vi "Run Tests in Test Case.vi"(8 "error in (no error)":errorcluster, 10 "Test Case":refnum<class "LUnit Test Case.lvclass">, 11 "Slave Test Runner In":refnum<class "Slave Test Runner.lvclass">) -> (0 "error out":errorcluster, 2 "Test Case out":refnum<class "LUnit Test Case.lvclass">, 3 "Slave Test Runner Out":refnum<class "Slave Test Runner.lvclass">)   [LabVIEW 2020, in "Slave Test Runner.lvclass"]
doc: "Run Methods in Test Case."
uses:
  Slave Test Runner.lvclass
  Test Case/LUnit Test Case.lvclass
  Test Case/LUnit Test Case.lvclass/LUnit Test Case.ctl
  Result Classes/Method Result/Method Result.lvclass/Method Result.ctl
  Result Classes/Test Case Result/Test Case Result.lvclass/Test Case Result.ctl
  Slave Test Runner.lvclass/Slave Test Runner.ctl
  Result Collector/Result Collector.lvclass/Result Collector.ctl
  Test Case/Private/SubVIs/Pre Allocate Method Results.vi
  Test Case/Public/Accessors/Read Enabled Test Methods.vi
  Shuffle Test Methods.vi/2fc74b80-6deb-4f17-a78e-34401938511c.vi
  Result Classes/Test Case Result/Community/Handle Error.vi
  Result Classes/Test Case Result/Community/Set Method End Time.vi
  Result Classes/Test Case Result/Public/Accessors/Read Method Results.vi
  Result Collector/Public/API/Collect Method Results.vi
  Result Collector/Public/API/Collect Case Result.vi
  Test Case/Private/SubVIs/Read Test Case Name.vi
  Result Classes/Test Case Result/Community/Preallocate Method Results.vi
  Result Classes/Method Result/Public/Read Status.vi
  Result Classes/Method Result/Community/Accessors/Generate Error.vi
  Result Classes/Method Result/Community/Accessors/Write Execution time.vi
  Result Classes/Method Result/Community/Accessors/Write Test Method Name.vi
  Result Classes/Method Result/Community/Accessors/Write Test Case.vi
  <vilib>/Utility/LVClass/Get LV Class Name.vi
  <vilib>/Utility/semaphor.llb/Obtain Semaphore Reference.vi
  <vilib>/Utility/error.llb/Error Cluster From Error Code.vi
  <vilib>/Utility/semaphor.llb/Release Semaphore Reference.vi
  Result Classes/Test Case Result/Test Case Result.lvclass
  Result Classes/Method Result/Method Result.lvclass
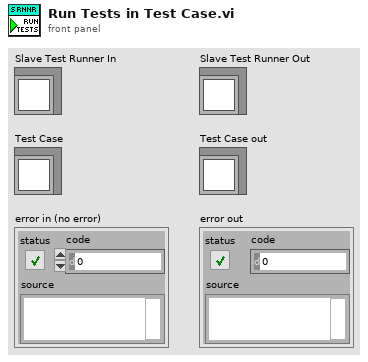
[diagram p1: front panel]
types:
  T1 = enum16{"Setup Error", "Teardown Error", "Broken", "Test Method Error"}
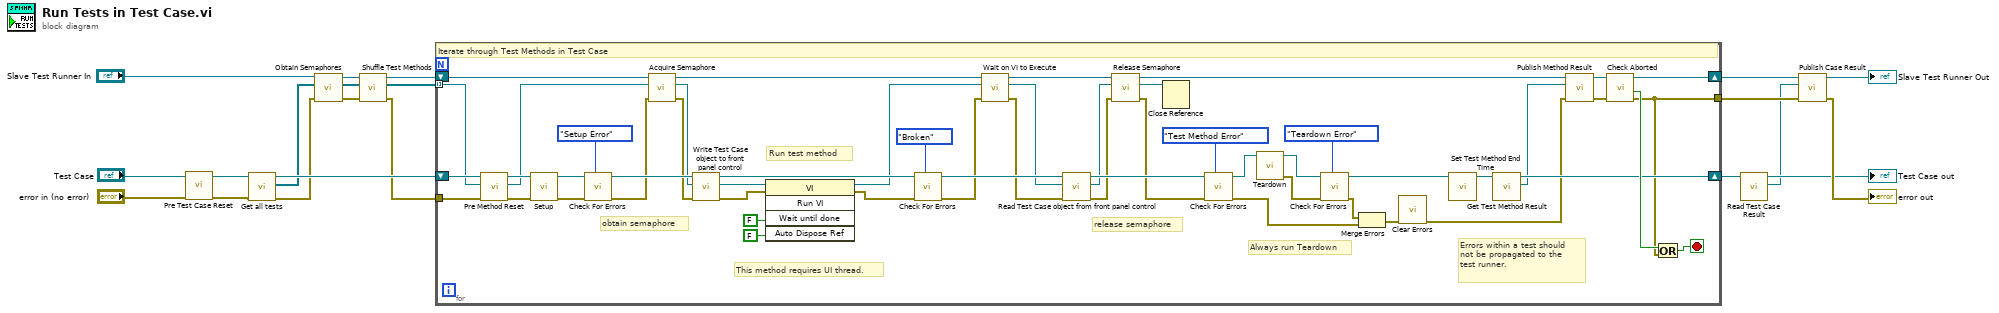
[diagram p0: block diagram]
diagram:
  n1 = call "Pre Test Case Reset.vi"("error in (no error)"="error in (no error)", "LUnit Test Case In"="Test Case") -> ("error out"=w15:errorcluster, "LUnit Test Case Out"=w16:refnum<class "LUnit Test Case.lvclass">)  [unwired: 8 in]
  n2 = call "Get all tests.vi"("error in (no error)"=w15, "Test Case in"=w16) -> ("error out"=w5:errorcluster, "VI refs out"=w7:refnum<vi>[], "Test Case out"=w19:refnum<class "LUnit Test Case.lvclass">)  [unwired: 7 in]
  n3 = call "Obtain Semaphores.vi"("error in (no error)"=w5, "VI refs in"=w7, "Slave Test Runner In"="Slave Test Runner In") -> ("error out"=w6:errorcluster, "VI Refs out"=w8:refnum<vi>[], "Slave Test Runner Out"=w9:refnum<class "Slave Test Runner.lvclass">)  [unwired: 6 in]
  n4 = call "Shuffle Test Methods.vi"("error in (no error)"=w6, "VI refs in"=w8, "Slave Test Runner in"=w9) -> ("error out"=w13:errorcluster, "shuffled array"=w12:refnum<vi>[], "Slave Test Runner out"=w11:refnum<class "Slave Test Runner.lvclass">)  [unwired: 6 in]
  n5 = for {
    tunnel: w12 -> [w35] mode=indexing
    shift-right: [w36] -> w4
    shift-left: w19 -> [w70]
    shift-right: [w53] -> w3
    shift-left: w11 -> [w51]
    tunnel: w13 -> [w68]
    tunnel: [w22] -> w2
    stop <- w23 stop-if-true
    # "This method requires UI thread."
    # "Run test method"
    # "release semaphore"
    # "obtain semaphore"
    # "Errors within a test should not be propagated to the test runner."
    # "Always run Teardown"
    # "Iterate through Test Methods in Test Case"
    n6 = call "Pre Method Reset.vi"("error in (no error)"=w68, "VI Refnum"=w35, "LUnit Test Case In"=w70) -> ("error out"=w69:errorcluster, "VI Refnum out"=w34:refnum<vi>, "LUnit Test Case Out"=w71:refnum<class "LUnit Test Case.lvclass">)  [unwired: 6 in]
    n7 = call-dynamic "Setup.vi"("error in (no error)"=w69, "LUnit Test Case In"=w71) -> ("error out"=w66:errorcluster, "LUnit Test Case Out"=w72:refnum<class "LUnit Test Case.lvclass">)  [unwired: 8 in]
    n8 = call "Check For Errors.vi"("Mode"=T1."Setup Error", "error in (no error)"=w66, "LUnit Test Case In"=w72) -> ("error out"=w47:errorcluster, "LUnit Test Case Out"=w67:refnum<class "LUnit Test Case.lvclass">)  [unwired: 7 in]
    n9 = call <vilib>:"Acquire Semaphore.vi"("error in (no error)"=w47, "VI Refnum in"=w34, "Slave Test Runner in"=w51) -> ("error out"=w46:errorcluster, "VI Refnum out"=w45:refnum<vi>, "Slave Test Runner out"=w48:refnum<class "Slave Test Runner.lvclass">)  [unwired: 6 in]
    n10 = call "Write Test Case object to front panel control.vi"("error in (no error)"=w46, "VI Refnum"=w45, "Test Case in"=w67) -> ("error out"=w73:errorcluster, "VI Refnum out"=w74:refnum<vi>, "Test Case out"=w63:refnum<class "LUnit Test Case.lvclass">)  [unwired: 6 in]
    n11 = invoke class="VI" method="Run VI"(reference=w74, error in=w73, "Wait until done"=FALSE ("Wait Until Done"), "Auto Dispose Ref"=FALSE ("Auto Dispose Reference")) -> (reference out=w33:refnum<vi>, error out=w38:errorcluster)  [unwired: 1 in, 3 out]
    n12 = call "Check For Errors.vi"("Mode"=T1."Broken", "error in (no error)"=w38, "LUnit Test Case In"=w63) -> ("error out"=w37:errorcluster, "LUnit Test Case Out"=w62:refnum<class "LUnit Test Case.lvclass">)  [unwired: 7 in]
    n13 = call "Wait on VI to Execute.vi"("error in (no error)"=w37, "VI Refnum in"=w33, "Slave Test Runner in"=w48) -> ("error out"=w49:errorcluster, "VI Refnum out"=w50:refnum<vi>, "Slave Test Runner out"=w44:refnum<class "Slave Test Runner.lvclass">)  [unwired: 6 in]
    n14 = call "Read Test Case object from front panel control.vi"("error in (no error)"=w49, "VI Refnum"=w50, "Test Case in"=w62) -> ("error out"=w42:errorcluster, "VI Refnum out"=w43:refnum<vi>, "Test Case out"=w61:refnum<class "LUnit Test Case.lvclass">)  [unwired: 6 in]
    n15 = call <vilib>:"Release Semaphore.vi"("error in (no error)"=w42, "VI in"=w43, "Slave Test Runner in"=w44) -> ("error out"=w32:errorcluster, "VI out"=w31:refnum<vi>, "Slave Test Runner out"=w28:refnum<class "Slave Test Runner.lvclass">)  [unwired: 6 in]
    n16 = Close Reference(reference=w31) -> ()  [unwired: 1 in, 1 out]
    n17 = call "Check For Errors.vi"("Mode"=T1."Test Method Error", "error in (no error)"=w32, "LUnit Test Case In"=w61) -> ("error out"=w54:errorcluster, "LUnit Test Case Out"=w60:refnum<class "LUnit Test Case.lvclass">)  [unwired: 7 in]
    n18 = call-dynamic "Teardown.vi"("LUnit Test Case In"=w60) -> ("error out"=w64:errorcluster, "LUnit Test Case Out"=w65:refnum<class "LUnit Test Case.lvclass">)  [unwired: 9 in]
    n19 = call "Check For Errors.vi"("Mode"=T1."Teardown Error", "error in (no error)"=w64, "LUnit Test Case In"=w65) -> ("error out"=w59:errorcluster, "LUnit Test Case Out"=w30:refnum<class "LUnit Test Case.lvclass">)  [unwired: 7 in]
    n20 = Merge Errors(w59, w54) -> (w55:errorcluster)
    n21 = call <vilib>:"Clear Errors.vi"("error in (no error)"=w55) -> ("error out"=w25:errorcluster)  [unwired: 5 in, 1 out]
    n22 = call "Set Test Method End Time.vi"("LUnit Test Case in"=w30) -> ("LUnit Test Case out"=w29:refnum<class "LUnit Test Case.lvclass">)  [unwired: 10 in]
    n23 = call "Get Test Method Result.vi"("LUnit Test Case In"=w29) -> ("Test Method Result"=w26:refnum<class "Method Result.lvclass">, "LUnit Test Case Out"=w36:refnum<class "LUnit Test Case.lvclass">)  [unwired: 9 in]
    n24 = call "Publish Method Result.vi"("error in (no error)"=w25, "Test Method Result"=w26, "Slave Test Runner In"=w28) -> ("error out"=w24:errorcluster, "Slave Test Runner Out"=w27:refnum<class "Slave Test Runner.lvclass">)  [unwired: 7 in]
    n25 = call "Check Aborted.vi"("error in (no error)"=w24, "Slave Test Runner In"=w27) -> ("error out"=w22:errorcluster, "Aborted?"=w52:bool, "Slave Test Runner Out"=w53:refnum<class "Slave Test Runner.lvclass">)  [unwired: 7 in]
    n26 = Or(x=w52, y=w22) -> (x .or. y?=w23:bool)
  }
  n27 = call "Read Test Case Result.vi"("LUnit Test Case In"=w4) -> ("Test Case Result"=w1:refnum<class "Test Case Result.lvclass">, "LUnit Test Case Out"=→"Test Case out":refnum<class "LUnit Test Case.lvclass">)  [unwired: 9 in]
  n28 = call "Publish Case Result.vi"("error in (no error)"=w2, "Test Case Result"=w1, "Slave Test Runner In"=w3) -> ("error out"=→"error out":errorcluster, "Slave Test Runner Out"=→"Slave Test Runner Out":refnum<class "Slave Test Runner.lvclass">)  [unwired: 7 in]
